vi "-Set Tuner Bandwidth.vi"(8 "error in (no error)":errorcluster, 10 "BandWidth":u32, 11 "RTL-SDR in":refnum<class "RTL-SDR.lvclass">) -> (0 "error out":errorcluster, 1 "function return":i32, 3 "RTL-SDR out":refnum<class "RTL-SDR.lvclass">)   [LabVIEW 2015, in "RTL-SDR.lvclass"]
doc: "Created IvanLis by LabVIEW Portal\nProfile: http://labviewportal.org/memberlist.php?mode=viewprofile&u=987\neMail: IvanLisanov@gMail.com\nTelegram: https://t.me/IvanLis"
uses:
  RTL-SDR.lvclass
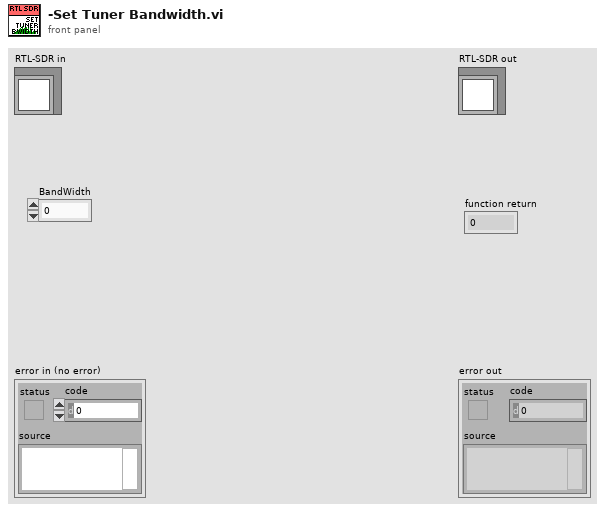
[diagram p1: front panel]
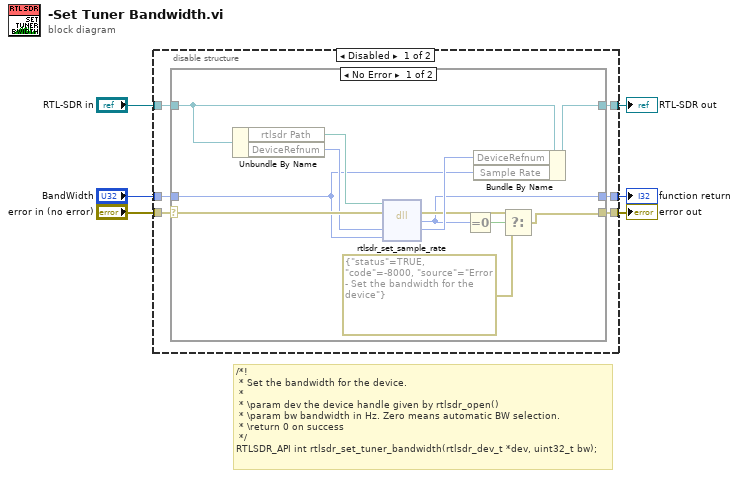
[diagram p0: block diagram]
diagram:
  # "/*!\n * Set the bandwidth for the device.\n *\n * \\param dev the device handle given by rtlsdr_open()\n * \\param bw bandwidth in Hz. Zero means automatic BW selection.\n * \\return 0 on success\n */\nRTLSDR_API int rtlsdr_set_tuner_bandwidth(rtlsdr_dev_t *dev, uint32_t bw);"
  n1 = disable-structure shown="Disabled" {
    disable-tunnel: "error in (no error)" -> [w12 w27]
    disable-tunnel: [w11 w27] -> w5
    disable-tunnel: "RTL-SDR in" -> [w10 w28]
    disable-tunnel: [w9 w28] -> w3
    disable-tunnel: [w8 _] -> w2
    disable-tunnel: "BandWidth" -> [w7 _]
    frame Disabled {
      n2 = case shown="No Error" w12 {
        selector: w12 -> [w24 w26]
        tunnel: [w14 w26] -> w11
        tunnel: [w20 w25] -> w9
        tunnel: w10 -> [w23 w25]
        tunnel: [w13 _] -> w8
        tunnel: w7 -> [w18 _]
        frame No Error {
          n3 = Unbundle By Name(w23) -> ("rtlsdr Path"=w21:path, "DeviceRefnum"=w22:u64)
          n4 = dll-call lib="C:/Users/Ivan/Desktop/D-23-09-24 (RTL-SDR)/Project (Pelleng-SDR)/rtlsdr/dll/rtlsdr.*" fn="rtlsdr_set_sample_rate"(path in=w21, error in=w24, "DeviceRefnum"=w22, "Sample Rate"=w18) -> (error out=w15:errorcluster, "return type"=w13:i32, "DeviceRefnum"=w19:u64)  [unwired: 2 in, 1 out]
          n5 = Equal To 0?(x=w13) -> (x = 0?=w17:bool)
          n6 = Bundle By Name(cluster=w23, "DeviceRefnum"=w19, "Sample Rate"=w18) -> (w20:refnum<class "RTL-SDR.lvclass">)
          n7 = Select(t=w15, s=w17, f=errorcluster {"status"=TRUE, "code"=-8000, "source"="Error - Set the bandwidth for the device"} ("error out")) -> (s? t:f=w14:errorcluster)
        }
        frame Error {
        }
      }
    }
    frame Enabled {
    }
  }
  "error out" <- w5
  "RTL-SDR out" <- w3
  "function return" <- w2
